vi "[GV]_GEAR.vi"() -> ()   [LabVIEW 2016]
panel:
  in  "GEAR":u16(ring) items=["Forward Drive", "Neutral", "Backward Drive"]
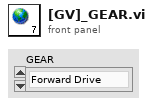
[diagram p1: front panel]
diagram:
